vi "Start.vi"(0 "eye scan in":refnum<class "niHighSpeedSerial Rectangular Eye Scan v1 Host.lvclass">, 11 "error in":errorcluster) -> (4 "eye scan out":refnum<class "niHighSpeedSerial Rectangular Eye Scan v1 Host.lvclass">, 15 "error out":errorcluster)   [LabVIEW 2014, in "niHighSpeedSerial Rectangular Eye Scan v1 Host.lvclass"]
doc: "Moves the session into the Running state and begins measuring the first point.\n\n<B>Input Parameters</B>\n\n<B>eye scan in</B> Takes in a reference to your session from the previous VI.\n\n<B>error in</B> describes error conditions that occur before this node runs. This input provides standard 'error in' functionality.\n\n<B>Output Parameters</B>\n\n<B>eye scan out</B> passes a reference to your session to the next VI.\n\n<B>error out</B> contains error information. This output provides standard 'error out' functionality."
uses:
  <instrlib>/niHighSpeedSerial/Eye Scan/v1/Host/Impl/Rectangular Eye Scan/niHighSpeedSerial Rectangular Eye Scan v1 Host.lvclass
  <instrlib>/niHighSpeedSerial/Eye Scan/v1/Host/Impl/Rectangular Eye Scan/niHighSpeedSerial Rectangular Eye Scan v1 Host.lvclass/niHighSpeedSerial Rectangular Eye Scan v1 Host.ctl
  <instrlib>/niHighSpeedSerial/Eye Scan/v1/Host/Eye Scan/niHighSpeedSerial Eye Scan v1 Host.lvclass
  <instrlib>/niHighSpeedSerial/Eye Scan/v1/Host/Impl/Rect Iter/niHighSpeedSerial Rectangular Eye Scan Point Iterator v1 Host.lvclass
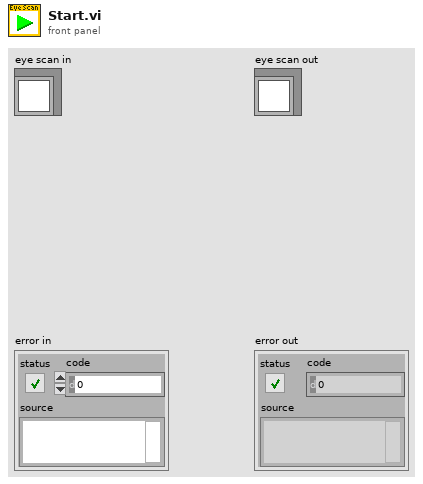
[diagram p1: front panel]
types:
  T1 = typedef "niHighSpeedSerial Eye Scan Common v1 Host.lvlib/RX Output Divider.ctl" = enum16{"1", "2", "4", "8", "16"}
  T2 = typedef "Rectangular Eye Scan v1 Host.lvclass/Private Data.ctl" = cluster{"horizontal step size":i16, "vertical step size":i16, "rectangular eye scan point iterator":refnum<class "niHighSpeedSerial Rectangular Eye Scan Point Iterator v1 Host.lvclass">}
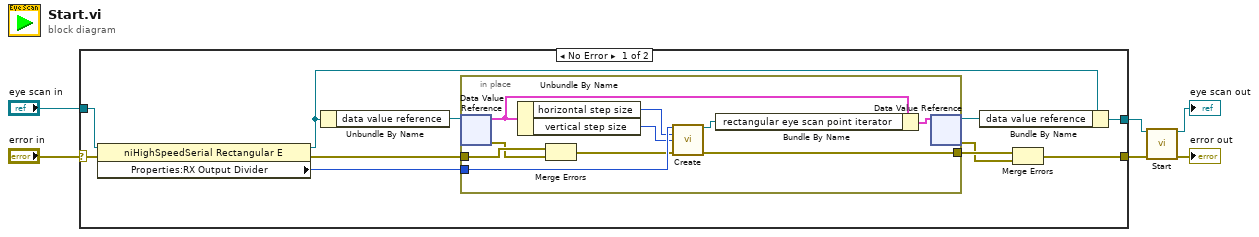
[diagram p0: block diagram]
diagram:
  n1 = case shown="No Error" "error in" {
    selector: "error in" -> [w7 w29]
    tunnel: [w16 w29] -> w1
    tunnel: [w17 w28] -> w2
    tunnel: "eye scan in" -> [w8 w28]
    frame No Error {
      n2 = property class="niHighSpeedSerial Rectangular E"(reference=w8, error in=w7) -> (reference out=w9:refnum<class "niHighSpeedSerial Rectangular Eye Scan v1 Host.lvclass">, error out=w14:errorcluster, "Properties:RX Output Divider"=w13:T1)
      n3 = Unbundle By Name(w9) -> ("data value reference"=w12:refnum<data-value>)
      n4 = in-place {
        in-place-border: [w27] -> w15
        in-place-border: w14 -> [w26]
        in-place-border: w13 -> [w25]
        n5 = in-place-dvr #1(w12) -> (w20:T2, w21:errorcluster)
        n6 = Unbundle By Name(w20) -> ("horizontal step size"=w23:i16, "vertical step size"=w22:i16)
        n7 = Merge Errors(w26, w21) -> (w24:errorcluster)
        n8 = call <instrlib>:"Create.vi"("rx output divider"=w25, "horizontal step size"=w23, "vertical step size"=w22, "error in"=w24) -> ("eye scan point iterator out"=w18:refnum<class "niHighSpeedSerial Rectangular Eye Scan Point Iterator v1 Host.lvclass">, "error out"=w27:errorcluster)  [unwired: 10 in]
        n9 = Bundle By Name(cluster=w20, "rectangular eye scan point iterator"=w18) -> (w19:T2)
        n10 = in-place-dvr #1(w19) -> (w11:refnum<data-value>, w10:errorcluster)
      }
      n11 = Bundle By Name(cluster=w9, "data value reference"=w11) -> (w17:refnum<class "niHighSpeedSerial Rectangular Eye Scan v1 Host.lvclass">)
      n12 = Merge Errors(w15, w10) -> (w16:errorcluster)
    }
    frame Error {
    }
  }
  n13 = call-parent "Start.vi"("eye scan in"=w2, "error in"=w1) -> ("eye scan out"=→"eye scan out":refnum<class "niHighSpeedSerial Rectangular Eye Scan v1 Host.lvclass">, "error out"=→"error out":errorcluster)  [unwired: 12 in]
